vi "Read Send Queue.vi"(8 "error in (no error)":errorcluster, 11 "send queue":refnum<queue>) -> (0 "error out":errorcluster, 3 "RESP3 Value":variant)   [LabVIEW 2019, in "Test Redis Client for LabVIEW.lvlib"]
uses:
  Test Redis Client for LabVIEW.lvlib
  lib/RESP3-for-LabVIEW/RESP3/RESP3 Parser/RESP3 Parser.lvclass
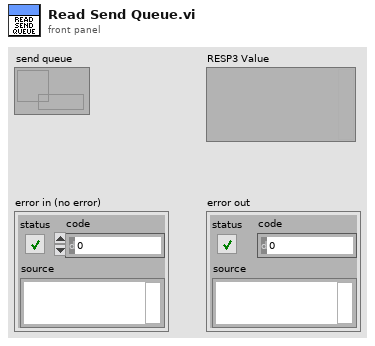
[diagram p1: front panel]
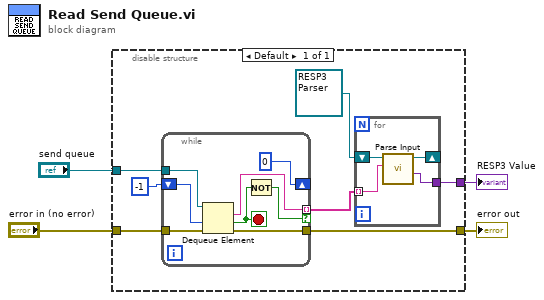
[diagram p0: block diagram]
diagram:
  n1 = disable-structure shown="Default" {
    disable-tunnel: [w11] -> w4
    disable-tunnel: [w7] -> w3
    disable-tunnel: "send queue" -> [w6]
    disable-tunnel: "error in (no error)" -> [w5]
    frame Enabled {
      n2 = while {
        tunnel: w6 -> [w23]
        tunnel: [w22] -> w10 mode=indexing if=w20
        tunnel: [w19] -> w7
        shift-right: [0 ("timeout in ms (-1)")] -> _
        shift-left: -1 ("timeout in ms (-1)") -> [w18]
        tunnel: w5 -> [w16]
        stop <- w21 stop-if-true
        n3 = Dequeue Element(queue=w23, timeout in ms (-1)=w18, error in (no error)=w16) -> (element=w22:string, timed out?=w21:bool, error out=w19:errorcluster)  [unwired: 1 out]
        n4 = Not(x=w21) -> (.not. x?=w20:bool)
      }
      n5 = for {
        shift-right: [w14] -> _
        shift-left: refnum<class "RESP3 Parser.lvclass"> refnum ("RESP3.lvlib:RESP3 Parser.lvclass") -> [w15]
        tunnel: [w13] -> w11
        tunnel: w10 -> [w12] mode=indexing
        n6 = call-dynamic "Parse Input.vi"("input line"=w12, "RESP3 Parser in"=w15) -> ("RESP3 Value"=w13:variant, "RESP3 Parser out"=w14:refnum<class "RESP3 Parser.lvclass">)  [unwired: 5 in, 3 out]
      }
    }
  }
  "RESP3 Value" <- w4
  "error out" <- w3
